vi "UDP example.vi"() -> ()   [LabVIEW 2012]
panel:
  out "Valid ?":bool
  in  "Tug letter":string="G"
  out "Buoy locations":cluster{"regular expression":string, i32, i32}[](array[cluster])
  out "Tug H":i32
  out "Tug Y":i32
  out "Tug X":i32
  in  "error in":errorcluster
  out "UDP Time Out?":bool
  out "data rec'd":string
  in  "stop":bool caption="ESTOP"
  # "Base station recieving code (example)"
  # "Type in L T G P  (look at boat cradle)"
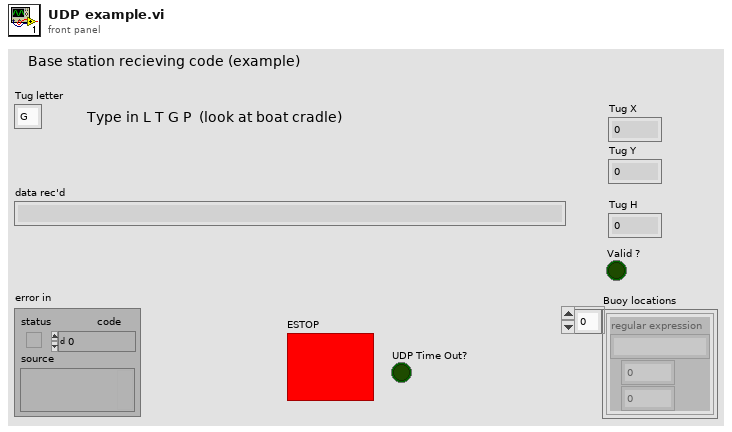
[diagram p1: front panel]
types:
  T1 = cluster{"regular expression":string, i32, i32, i32}
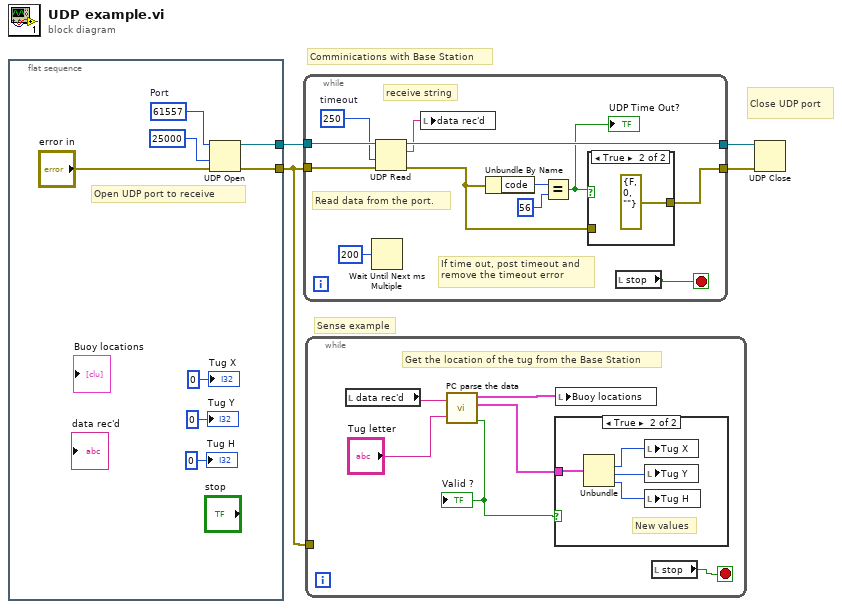
[diagram p0: block diagram]
diagram:
  # "Sense example"
  # "Comminications with Base Station"
  # "Close UDP port"
  n1 = flat-sequence {
    tunnel: [w10] -> w2
    tunnel: [w9] -> w1
    frame #0 {
      w12 = u16 61557  # Port
      # "Open UDP port to receive"
      n2 = UDP Open(8:"error in", 9:25000 ("timeout ms (25000)"), 11:w12) -> (port=w10:refnum<k16>, 0:w9:errorcluster)  [unwired: 2 in, 1 out]
      "Tug X" <- 0 ("Tug X")
      "Tug Y" <- 0 ("Tug Y")
      "Tug H" <- 0 ("Tug H")
    }
  }
  n3 = while {
    tunnel: w1 -> [w24]
    tunnel: w2 -> [w23]
    tunnel: [w22] -> w4
    tunnel: [w17] -> w3
    stop <- w13 stop-if-true
    w16 = 250  # timeout
    # "receive string"
    # "If time out, post timeout and\nremove the timeout error"
    # "Read data from the port."
    n4 = Wait Until Next ms Multiple(millisecond multiple=u32 200) -> ()  [unwired: 1 out]
    n5 = UDP Read(connection ID=w23, timeout ms (25000)=w16, 8:w24) -> (data out=w15:string, error out=w18:errorcluster, 3:w22:refnum<k16>)  [unwired: 1 in, 2 out]
    n6 = local write "data rec'd"(w15) -> ()
    n7 = Unbundle By Name(w18) -> ("code"=w21:i32)
    n8 = Equal?(x=w21, y=56) -> (x = y?=w19:bool)
    "UDP Time Out?" <- w19
    n9 = case shown="True" w19 {
      tunnel: [w25 errorcluster {"status"=FALSE, "code"=0, "source"=""} ("error out")] -> w17
      tunnel: w18 -> [w25 _]
      frame False {
      }
      frame True {
      }
    }
    n10 = local read "stop"() -> (w13:bool)
  }
  n11 = while {
    tunnel: w1 -> [_]
    stop <- w27 stop-if-true
    # "Get the location of the tug from the Base Station"
    n12 = local read "data rec'd"() -> (w32:string)
    n13 = call "PC parse the data.vi"("Nav String"=w32, "Tug"="Tug letter") -> ("Buoy locations"=w28:cluster{"regular expression":string, i32, i32}[], "Tug Location"=w30:T1, "Valid?"=w29:bool)  [unwired: 1 out]
    "Valid ?" <- w29
    n14 = case shown="True" w29 {
      tunnel: w30 -> [_ w36]
      frame False {
        # "No \nchange"
      }
      frame True {
        # "New values"
        n15 = Unbundle(w36) -> (w35:i32, w34:i32, w33:i32)  [unwired: 1 out]
        n16 = local write "Tug X"(w35) -> ()
        n17 = local write "Tug Y"(w34) -> ()
        n18 = local write "Tug H"(w33) -> ()
      }
    }
    n19 = local write "Buoy locations"(w28) -> ()
    n20 = local read "stop"() -> (w27:bool)
  }
  n21 = UDP Close(connection ID=w4, 8:w3) -> ()  [unwired: 2 out]
